vi "CheckIfEventRead.vi"(8 "error in (no error)":errorcluster, 10 "Read?":refnum<notifier>) -> (0 "error out":errorcluster, 2 "Read":bool)   [LabVIEW 2019, in "Setting Database.lvclass"]
uses:
  Setting Database.lvclass
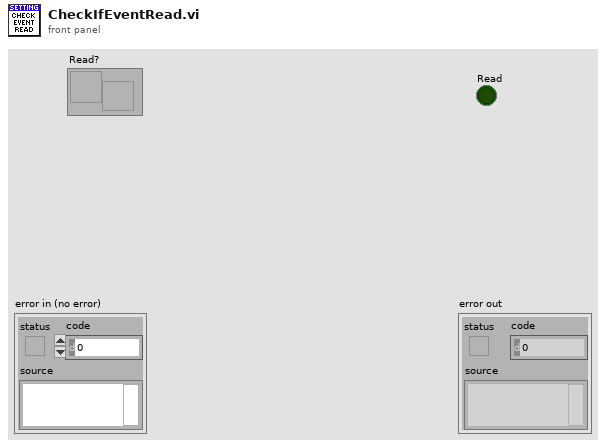
[diagram p1: front panel]
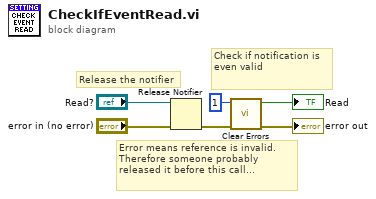
[diagram p0: block diagram]
diagram:
  # "Error means reference is invalid. Therefore someone probably released it before this call..."
  # "Check if notification is even valid"
  # "Release the notifier"
  n1 = Release Notifier(notifier="Read?", error in (no error)="error in (no error)") -> (error out=w3:errorcluster)  [unwired: 1 in, 2 out]
  n2 = call <vilib>:"Clear Errors.vi"("error in (no error)"=w3, "specific error code to clear (0: all)"=1) -> ("error out"=→"error out":errorcluster, "specific error cleared?"=→"Read":bool)  [unwired: 4 in]
